vi "TDMS.GetChannelsForLevelTransitionAnalysis.vi"(8 "error in (no error)":errorcluster, 11 "TDMS Ref":refnum<k34>) -> (0 "error out":errorcluster, 1 "ODH Channels":string[](array[string]), 2 "OPH Channels":string[](array[string]), 3 "TDMS Ref out":refnum<k34>)   [LabVIEW 2015, in "TestStand Analysis Steps.lvlib"]
uses:
  TestStand Analysis Steps.lvlib
  Shared/Constants.vi
  Shared/Shared.lvlib
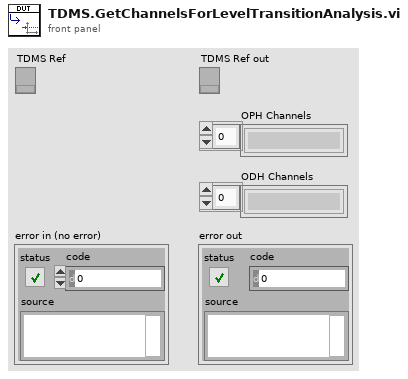
[diagram p1: front panel]
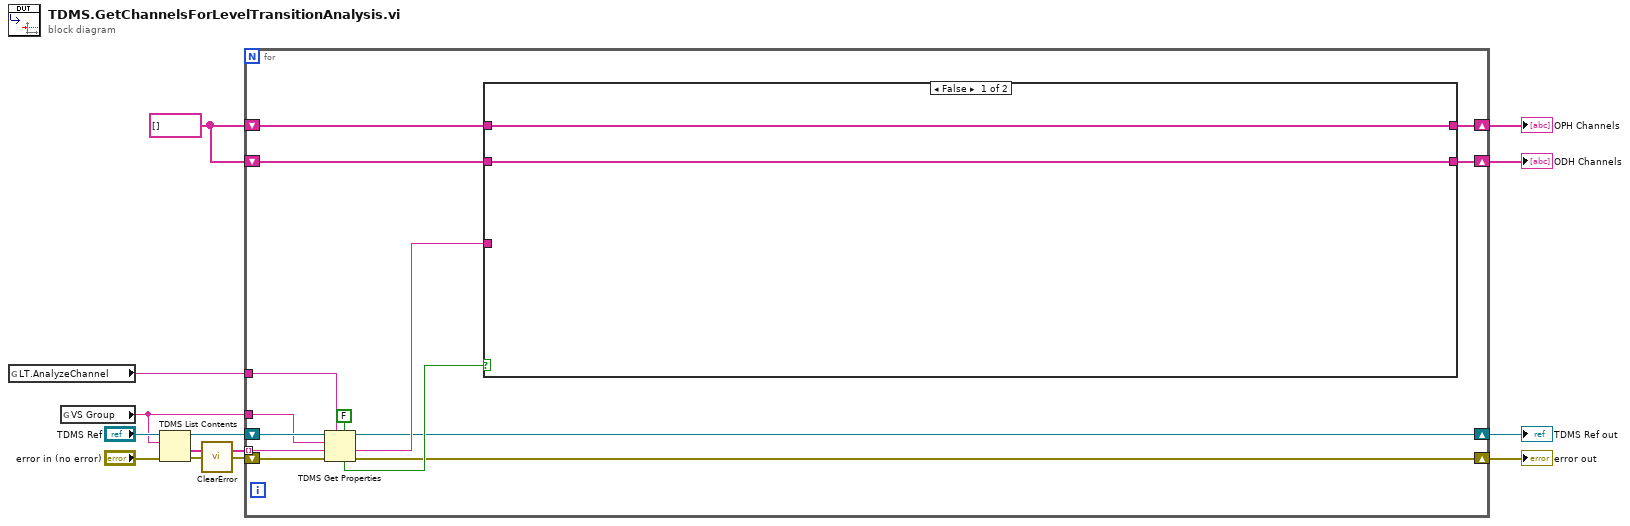
[diagram p0: block diagram]
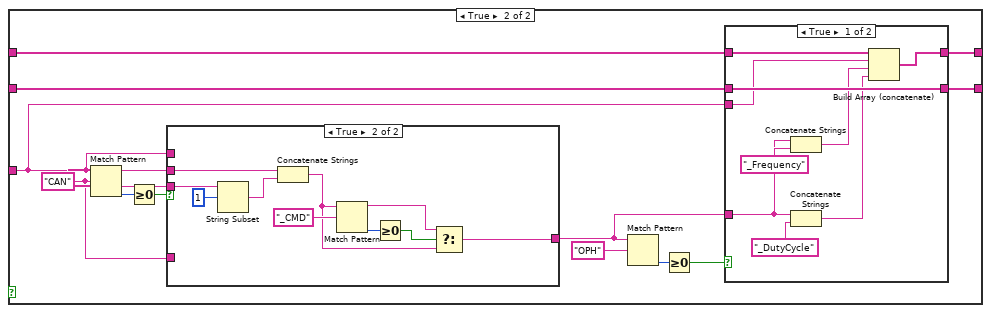
[diagram p2: hidden frame]
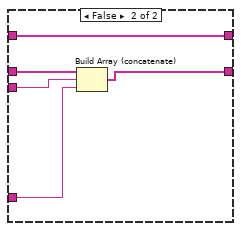
[diagram p3: hidden frame]
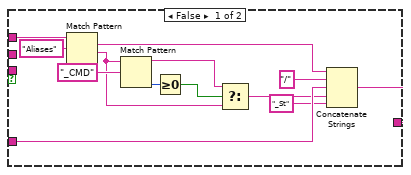
[diagram p4: hidden frame]
diagram:
  w9 = string[] []
  n1 = global read "Constants.vi" "LT.AnalyzeChannel"() -> (w1:string)
  n2 = global read "Constants.vi" "VS Group"() -> (w2:string)
  n3 = TDMS List Contents(4:"error in (no error)", 6:w2, 7:"TDMS Ref") -> (0:w3:errorcluster, 1:w8:string[], 3:w6:refnum<k34>)  [unwired: 1 out]
  n4 = call <vilib>:"ClearError.vi"("error in (no error)"=w3) -> ("error out"=w4:errorcluster)
  n5 = for {
    shift-right: [w24] -> w11
    shift-left: w9 -> [w27]
    shift-right: [w25] -> w10
    shift-left: w9 -> [w26]
    tunnel: w8 -> [w22] mode=indexing
    shift-right: [w18] -> w12
    shift-left: w6 -> [w19]
    shift-right: [w16] -> w13
    shift-left: w4 -> [w17]
    tunnel: w2 -> [w15]
    tunnel: w1 -> [w14]
    n6 = TDMS Get Properties(5:FALSE, 7:w14, 8:w17, 9:w22, 10:w15, 11:w19) -> (0:w16:errorcluster, 1:w20:string, 3:w18:refnum<k34>, 4:w21:bool)  [unwired: 2 out]
    n7 = case shown="False" w21 {
      tunnel: w20 -> [_ w30]
      tunnel: w27 -> [w29 w34]
      tunnel: w26 -> [w28 w33]
      tunnel: [w28 w32] -> w25
      tunnel: [w29 w31] -> w24
      frame False {
      }
      frame True {
        w39 = "CAN" ("regular expression")
        n8 = Match Pattern(string=w30, regular expression=w39) -> (before substring=w41:string, after substring=w40:string, offset past match=w43:i32)  [unwired: 1 in, 1 out]
        n9 = Greater Or Equal To 0?(x=w43) -> (x >= 0?=w42:bool)
        n10 = case shown="True" w42 {
          tunnel: w41 -> [_ w77]
          tunnel: w40 -> [_ w79]
          tunnel: [w65 w71] -> w36
          tunnel: w30 -> [w70 _]
          tunnel: w39 -> [w68 _]
          frame False {
            n11 = Match Pattern(string=w70, regular expression="Aliases") -> (match substring=w66:string, after substring=w59:string)  [unwired: 1 in, 2 out]
            n12 = Match Pattern(string=w59, regular expression="_CMD") -> (before substring=w60:string, offset past match=w62:i32)  [unwired: 1 in, 2 out]
            n13 = Greater Or Equal To 0?(x=w62) -> (x >= 0?=w61:bool)
            n14 = Select(t=w60, s=w61, f=w59) -> (s? t:f=w58:string)
            n15 = Concatenate Strings(w66, "/" ("string"), w68, w58, "_St" ("string")) -> (w65:string)
          }
          frame True {
            n16 = String Subset(string=w79, offset (0)=1) -> (substring=w78:string)  [unwired: 1 in]
            n17 = Concatenate Strings(w77, w78) -> (w72:string)
            n18 = Match Pattern(string=w72, regular expression="_CMD") -> (before substring=w73:string, offset past match=w75:i32)  [unwired: 1 in, 2 out]
            n19 = Greater Or Equal To 0?(x=w75) -> (x >= 0?=w74:bool)
            n20 = Select(t=w73, s=w74, f=w72) -> (s? t:f=w71:string)
          }
        }
        n21 = Match Pattern(string=w36, regular expression="OPH") -> (offset past match=w37:i32)  [unwired: 1 in, 3 out]
        n22 = Greater Or Equal To 0?(x=w37) -> (x >= 0?=w35:bool)
        n23 = case shown="True" w35 {
          tunnel: w36 -> [w50 w56]
          tunnel: w30 -> [w47 w57]
          tunnel: w34 -> [w48 w53]
          tunnel: w33 -> [w49 w55]
          tunnel: [w49 w54] -> w32
          tunnel: [w44 w53] -> w31
          frame True {
            n24 = Concatenate Strings(w50, "_Frequency" ("string")) -> (w46:string)
            n25 = Concatenate Strings(w50, "_DutyCycle" ("string")) -> (w45:string)
            n26 = Build Array (concatenate)(w48, w47, w46, w45) -> (w44:string[])
          }
          frame False {
            n27 = Build Array (concatenate)(w55, w57, w56) -> (w54:string[])
          }
        }
      }
    }
  }
  "error out" <- w13
  "TDMS Ref out" <- w12
  "OPH Channels" <- w11
  "ODH Channels" <- w10
